vi "AI Main Page.vi"(8 "error in (no error)":errorcluster, 11 "Node Ptr":T1 format="%.0x") -> (0 "error out":errorcluster)   [LabVIEW 2013]
uses:
  <vilib>/K2Labs/HiLab API/Custom Device API/Controls/Custom Device Item Reference.ctl
  <vilib>/K2Labs/HiLab API/Custom Device API/Custom Device API Library.lvlib
panel:
  in  "Import":bool
  in  "NAME":string caption="Name"
  in  "DESCRIPTION":string caption="Description"
  in  "Channel List":i32(listbox)
  # "Analog Input"
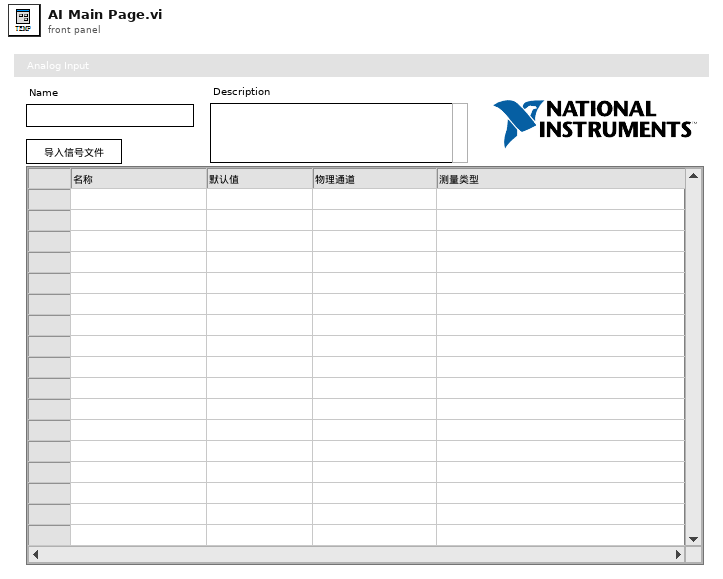
[diagram p1: front panel]
types:
  T1 = typedef "Custom Device API Library.lvlib/Custom Device Item Reference.ctl" = u64
  T2 = typedef "Custom Device API Library.lvlib/Custom Device System Configuration Command Type.ctl" = enum16{"Default", "Menu Selected", "Shutdown", "Dynamic button pressed"}
  T3 = typedef "AI Param.ctl" = cluster{"Name":string, "Description":string, "DefaultValue":dbl, "Physical Channel":string, "MeasurementType":T4, "Max":dbl, "Min":dbl, "Terminal Configuration":T5, "Units":string}
  T4 = typedef "MeasurementType.ctl" = enum16{"Voltage", "Current", "More:Voltage:Custom with Excitation", "More:Current:Custom with Excitation", "Frequency", "Period", "Resistance", "Temperature:Thermocouple", "Temperature:Thermistor", "Temperature:RTD", "Temperature:Built-in Sensor", "Strain Gage"}
  T5 = typedef "AI Terminal Configuration.ctl" = enum16{"默认", "RSE", "NRSE", "差分", "伪差分"}
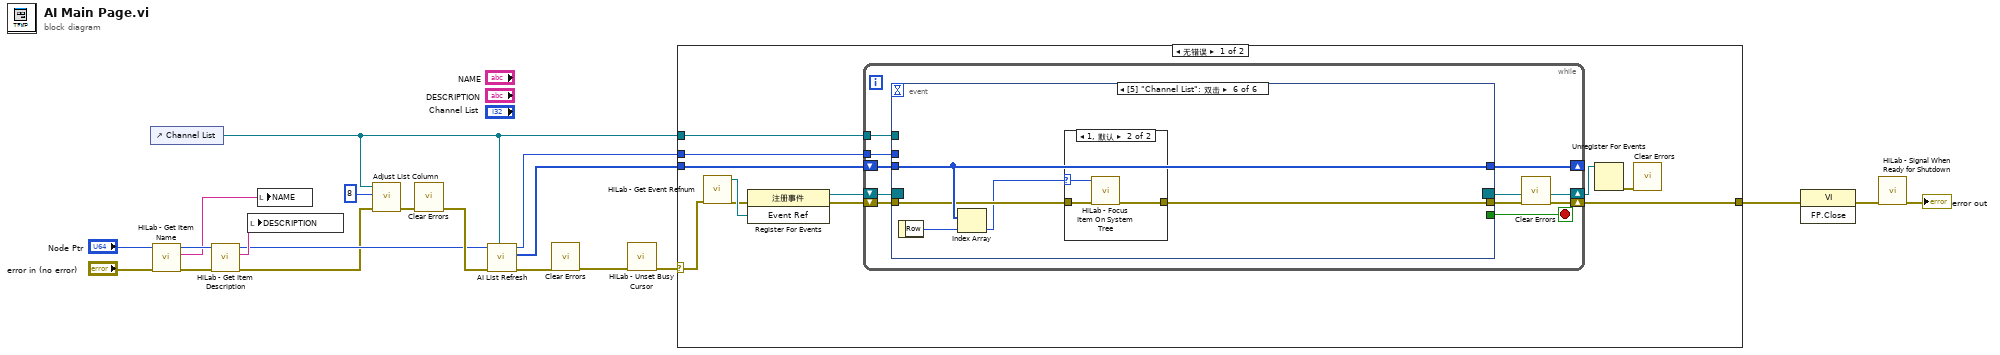
[diagram p0: block diagram]
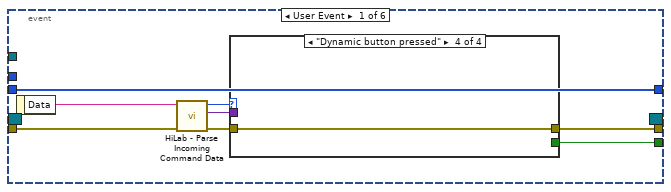
[diagram p2: hidden frame]
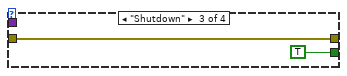
[diagram p5: hidden frame]
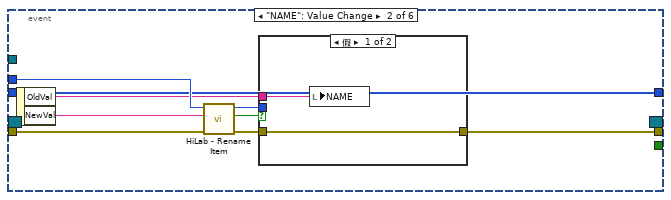
[diagram p6: hidden frame]
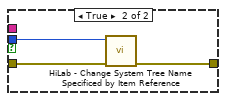
[diagram p7: hidden frame]
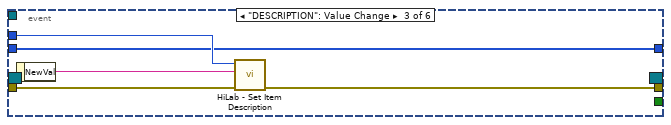
[diagram p8: hidden frame]
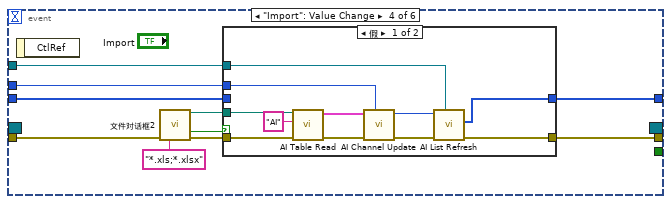
[diagram p9: hidden frame]
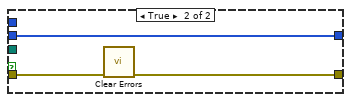
[diagram p10: hidden frame]
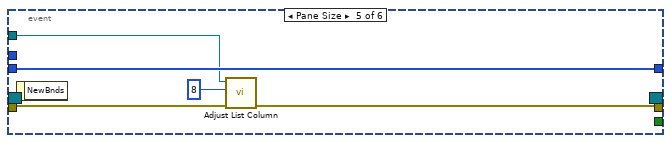
[diagram p11: hidden frame]
diagram:
  n1 = control-ref of="Channel List"() -> (w1:refnum<vi>)
  n2 = call <vilib>:"HiLab - Get Item Name.vi"("error in (no error)"="error in (no error)", "Item Ref in"="Node Ptr") -> ("error out"=w19:errorcluster, "Name"=w17:string, "Item Ref out"=w20:T1)  [unwired: 6 in, 1 out]
  n3 = call <vilib>:"HiLab - Get Item Description.vi"("error in (no error)"=w19, "Item Ref in"=w20) -> ("error out"=w7:errorcluster, "Discription"=w18:string, "Item Ref out"=w8:T1)  [unwired: 6 in, 1 out]
  n4 = local write "DESCRIPTION"(w18) -> ()
  n5 = local write "NAME"(w17) -> ()
  n6 = call "Adjust List Column.vi"("error in (no error)"=w7, "Column"=8, "MCListBox in"=w1) -> ("error out"=w10:errorcluster)  [unwired: 7 in, 1 out]
  n7 = call <vilib>:"Clear Errors.vi"("error in (no error)"=w10) -> ("error out"=w9:errorcluster)  [unwired: 6 in]
  n8 = call "AI List Refresh.vi"("VarList"=w1, "错误输入（无错误）"=w9, "Device Ref in"=w8) -> ("error out"=w6:errorcluster, "Channel Refs"=w3:T1[], "Device Ref out"=w4:T1)  [unwired: 6 in]
  n9 = call <vilib>:"Clear Errors.vi"("error in (no error)"=w6) -> ("error out"=w5:errorcluster)  [unwired: 6 in]
  n10 = call <vilib>:"HiLab - Unset Busy Cursor.vi"("error in (no error)"=w5) -> ("error out"=w13:errorcluster)  [unwired: 10 in]
  n11 = case shown="无错误" w13 {
    selector: w13 -> [w23 w111]
    tunnel: [w31 w111] -> w16
    tunnel: w4 -> [w30 _]
    tunnel: w1 -> [w22 _]
    tunnel: w3 -> [w21 _]
    frame No Error {
      n12 = call <vilib>:"HiLab - Get Event Refnum.vi"("error in (no error)"=w23) -> ("error out"=w25:errorcluster, "Event Ref"=w26:refnum<user-event>)  [unwired: 9 in]
      n13 = register-events(error in=w25, w26) -> (reference out=w29:refnum<event-registration>, error out=w27:errorcluster)  [unwired: 1 in]
      n14 = while {
        shift-right: [w40] -> w31
        shift-left: w27 -> [w41]
        tunnel: w30 -> [w39]
        shift-right: [w37] -> w28
        shift-left: w29 -> [w38]
        tunnel: w22 -> [w34]
        shift-right: [w32] -> _
        shift-left: w21 -> [w33]
        stop <- w36 stop-if-true
        n15 = event shown="[5] \"Channel List\": 双击" {
          selector: w38 -> [_ _ _ _ _ _]
          dyn-events: [_ _ _ _ _ _] -> w37
          timeout: _ -> [_ _ _ _ _ _]
          tunnel: [w44 _ _ _ _ _] -> w36
          tunnel: w41 -> [w48 w62 w72 w79 w101 w104]
          tunnel: [w45 w56 w70 w74 w100 w103] -> w35
          tunnel: w39 -> [_ w63 w73 w78 _ _]
          tunnel: w34 -> [_ _ _ w77 w97 _]
          tunnel: w33 -> [w42 w55 w69 w75 w99 w106]
          tunnel: [w42 w55 w69 w76 w99 w106] -> w32
          event User Event {
            n16 = event-data() -> ("Data"=w49:string)  [unwired: 1 in]
            n17 = call <vilib>:"HiLab - Parse Incoming Command Data.vi"("error in (no error)"=w48, "Incoming Command Data"=w49) -> ("error out"=w46:errorcluster, "Data"=w43:variant, "Actions"=w47:T2)  [unwired: 7 in]
            n18 = case shown="\"Dynamic button pressed\"" w47 {
              tunnel: w46 -> [w50 w51 w52 w54]
              tunnel: [w50 w51 w52 w54] -> w45
              tunnel: [_ _ TRUE _] -> w44
              tunnel: w43 -> [_ _ _ _]
              frame "Default", Default {
              }
              frame "Menu Selected" {
              }
              frame "Shutdown" {
              }
              frame "Dynamic button pressed" {
              }
            }
          }
          event "NAME": Value Change {
            n19 = event-data() -> ("OldVal"=w59:string, "NewVal"=w61:string)  [unwired: 1 in]
            n20 = call <vilib>:"HiLab - Rename Item.vi"("error in (no error)"=w62, "New Name"=w61, "Item Ref in"=w63) -> ("error out"=w57:errorcluster, "Success?"=w60:bool, "Item Ref out"=w58:T1)  [unwired: 6 in]
            n21 = case shown="假" w60 {
              tunnel: w59 -> [w65 _]
              tunnel: w58 -> [_ w68]
              tunnel: w57 -> [w64 w67]
              tunnel: [w64 w66] -> w56
              frame False {
                n22 = local write "NAME"(w65) -> ()
              }
              frame True {
                n23 = call <vilib>:"HiLab - Change System Tree Name Specificed by Item Reference.vi"("error in (no error)"=w67, "Item Ref in"=w68) -> ("error out"=w66:errorcluster)  [unwired: 8 in, 1 out]
              }
            }
          }
          event "DESCRIPTION": Value Change {
            n24 = event-data() -> ("NewVal"=w71:string)  [unwired: 1 in]
            n25 = call <vilib>:"HiLab - Set Item Description.vi"("error in (no error)"=w72, "Discription"=w71, "Item Ref in"=w73) -> ("error out"=w70:errorcluster)  [unwired: 6 in, 2 out]
          }
          event "Import": Value Change {
            n26 = event-data() -> ()  [unwired: 1 in, 1 out]
            n27 = call "文件对话框2"("error in"=w79, "pattern (all files)"="*.xls;*.xlsx") -> ("selected path"=w83:path, "cancelled"=w81:bool, "error out"=w82:errorcluster)  [unwired: 10 in, 1 out]
            n28 = case shown="假" w81 {
              tunnel: w82 -> [w91 w96]
              tunnel: w83 -> [w93 _]
              tunnel: [w86 w95] -> w74
              tunnel: w78 -> [w88 _]
              tunnel: w77 -> [w85 _]
              tunnel: [w84 w94] -> w76
              tunnel: w75 -> [_ w94]
              frame False {
                n29 = call "AI Table Read.vi"("error in (no error)"=w91, "Task"="AI", "Read Path"=w93) -> ("error out"=w89:errorcluster, "TaskParam"=w90:T3[])  [unwired: 5 in, 2 out]
                n30 = call "AI Channel Update.vi"("Device Ref"=w88, "error in (no error)"=w89, "DIChannel"=w90) -> ("error out"=w87:errorcluster)  [unwired: 8 in]
                n31 = call "AI List Refresh.vi"("VarList"=w85, "错误输入（无错误）"=w87, "Device Ref in"=w88) -> ("error out"=w86:errorcluster, "Channel Refs"=w84:T1[])  [unwired: 6 in, 1 out]
              }
              frame True {
                n32 = call <vilib>:"Clear Errors.vi"("error in (no error)"=w96) -> ("error out"=w95:errorcluster)  [unwired: 6 in]
              }
            }
          }
          event Pane Size {
            n33 = event-data() -> ()  [unwired: 1 in, 1 out]
            n34 = call "Adjust List Column.vi"("error in (no error)"=w101, "Column"=8, "MCListBox in"=w97) -> ("error out"=w100:errorcluster)  [unwired: 7 in, 1 out]
          }
          event "Channel List": Double Click {
            n35 = event-data() -> ("Row"=w105:i32)  [unwired: 1 in]
            n36 = Index Array(array=w106, index=w105) -> (element=w102:T1)
            n37 = case shown="1, 默认" w102 {
              selector: w102 -> [_ w108]
              tunnel: w104 -> [w107 w110]
              tunnel: [w107 w109] -> w103
              frame 0 {
              }
              frame 1, Default {
                n38 = call <vilib>:"HiLab - Focus Item On System Tree.vi"("error in (no error)"=w110, "Item Ref in"=w108) -> ("error out"=w109:errorcluster)  [unwired: 8 in, 1 out]
              }
            }
          }
        }
        n39 = call <vilib>:"Clear Errors.vi"("error in (no error)"=w35) -> ("error out"=w40:errorcluster)  [unwired: 6 in]
      }
      n40 = Unregister For Events(event registration refnum=w28) -> (error out=w24:errorcluster)  [unwired: 1 in]
      n41 = call <vilib>:"Clear Errors.vi"("error in (no error)"=w24) -> ()  [unwired: 6 in, 1 out]
    }
    frame Error {
    }
  }
  n42 = invoke class="VI" method="FP.Close"(error in=w16) -> (error out=w15:errorcluster)  [unwired: 2 in, 2 out]
  n43 = call <vilib>:"HiLab - Signal When Ready for Shutdown.vi"("error in (no error)"=w15) -> ("error out"=→"error out":errorcluster)  [unwired: 10 in]
